vi "sterownik.vi"() -> ()   [LabVIEW 2020]
uses:
  <vilib>/Platform/TimedLoop/XDataNode/timing_clust.ctl
  <vilib>/Platform/TimedLoop/XDataNode/nitl_modes.ctl
  <vilib>/Platform/TimedLoop/XDataNode/wakeup.ctl
  <vilib>/Platform/TimedLoop/XDataNode/XDataNode.xnode
  <vilib>/Platform/TimedLoop/XDataNode/XDNodeRunTimeDep.lvlib
panel:
  in  "histereza":dbl
  in  "h2max":dbl
  in  "h2min":dbl
  in  "h1max":dbl
  in  "h1min":dbl
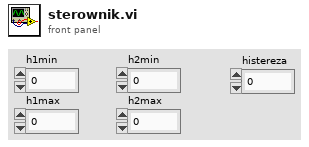
[diagram p1: front panel]
types:
  T1 = typedef "XDNodeRunTimeDep.lvlib/timing_clust.ctl" = cluster{"Expected End [f-1]":u64, "Actual End [f-1]":u64, "Finished Late? [f-1]":bool, "Expected End [i-1]":u64, "Actual End [i-1]":u64, "Finished Late? [i-1]":bool, "Expected Start [i]":u64, "Actual Start [i]":u64, "Expected Start [f]":u64, "Actual Start [f]":u64, "Source Name":string, "Structure Name":string, "Period":i64, "Deadline":i64, "Offset":i64, "Start":i64, "Priority":i32, "Timeout":i32, "Mode":T2, "Wakeup Reason":T3, "Error":errorcluster, "Source Type":string, "Secondary Source Type":string, "Global End Time":u64, "Global Start Time":u64, "Frame Duration":u64, "Iteration Duration":u64, "Assigned CPU":i32, "I/O Scan Engine Mode":u32}
  T2 = typedef "XDNodeRunTimeDep.lvlib/nitl_modes.ctl" = enum32{"No Change", "Process missed periods, maintain original phase", "Discard missed periods, maintain original phase", "Process missed periods, ignore original phase", "Discard missed periods, ignore original phase"}
  T3 = typedef "XDNodeRunTimeDep.lvlib/wakeup.ctl" = enum32{"Normal", "Aborted", "Asynchronous wakeup", "Timing source error", "Timed loop error", "Timeout"}
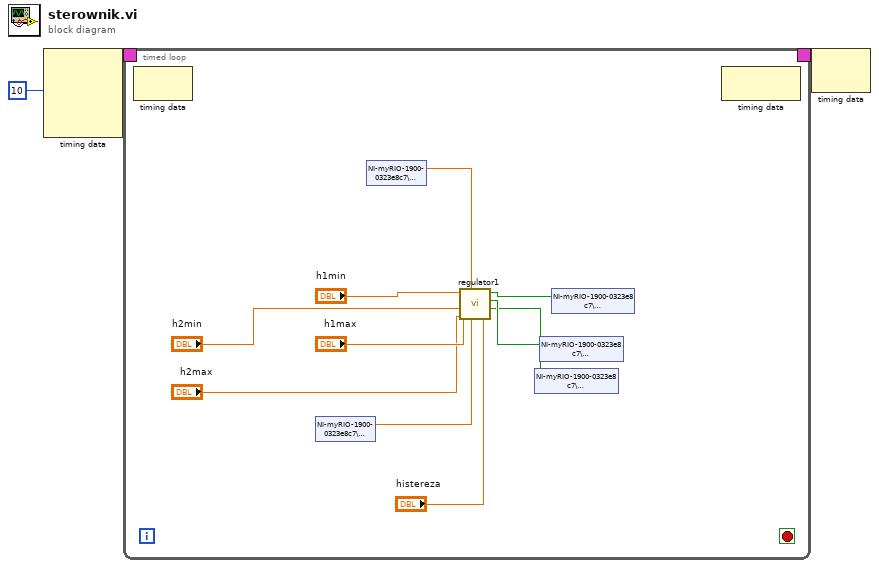
[diagram p0: block diagram]
diagram:
  n1 = node-c288(i64 10 ("Period")) -> (w3:T1)  [unwired: 3 in]
  n2 = timed-loop {
    timing: w3 -> [_]
    timing-out: [_] -> w2
    stop <- _ stop-if-true
    n3 = node-c288() -> ()  [unwired: 1 in, 1 out]
    n4 = shared-variable "NI-myRIO-1900-0323e8c7\\zmienneWspoldzielone.lvlib\\H2"() -> (w8:dbl)  [unwired: 1 in, 1 out]
    n5 = shared-variable "NI-myRIO-1900-0323e8c7\\zmienneWspoldzielone.lvlib\\H1"() -> (w12:dbl)  [unwired: 1 in, 1 out]
    n6 = call "regulator1.vi"("histereza"="histereza", "H2 [cm]"=w8, "H1 [cm]"=w12, "h2max"="h2max", "h2min"="h2min", "h1max"="h1max", "h1min"="h1min") -> ("Zawor2"=w9:bool, "Zawor1"=w10:bool, "Pompa"=w11:bool)
    n7 = shared-variable "NI-myRIO-1900-0323e8c7\\zmienneWspoldzielone.lvlib\\Zawor2"(w9) -> ()  [unwired: 1 in, 1 out]
    n8 = shared-variable "NI-myRIO-1900-0323e8c7\\zmienneWspoldzielone.lvlib\\Zawor1"(w10) -> ()  [unwired: 1 in, 1 out]
    n9 = shared-variable "NI-myRIO-1900-0323e8c7\\zmienneWspoldzielone.lvlib\\Pompa"(w11) -> ()  [unwired: 1 in, 1 out]
    n10 = node-c288() -> ()  [unwired: 1 in, 1 out]
  }
  n11 = node-c288(w2) -> ()  [unwired: 1 out]
